vi "Init2DListCtrl.vi"(8 "align":enum16{"Left", "Center", "Right"}(ring), 9 "background color":u32(colorbox)=16777226, 10 "type":enum16{"left frame", "top frame", "content"}(ring), 11 "ArrayRef in":refnum<vi>) -> (3 "ArrayRef out":refnum<vi>)   [LabVIEW 2018, in "Library-Ctrl.lvlib"]
uses:
  Library-Ctrl.lvlib
  <vilib>/Utility/miscctls.llb/LVRowAndColumnTypeDef.ctl
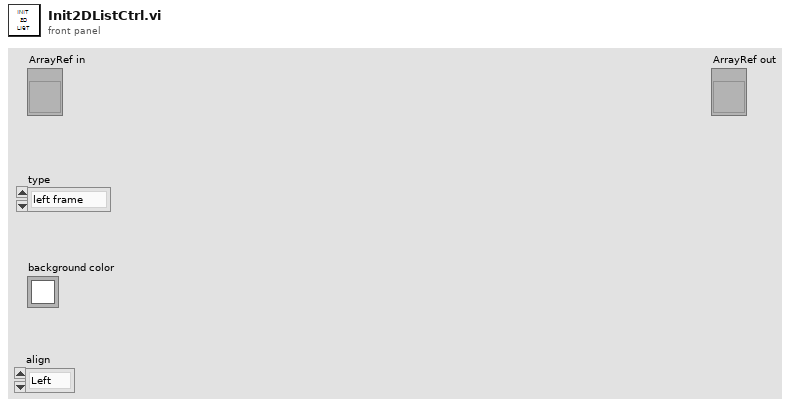
[diagram p1: front panel]
types:
  T1 = typedef "LVRowAndColumnTypeDef.ctl" = cluster{"Row":i32, "Column":i32}
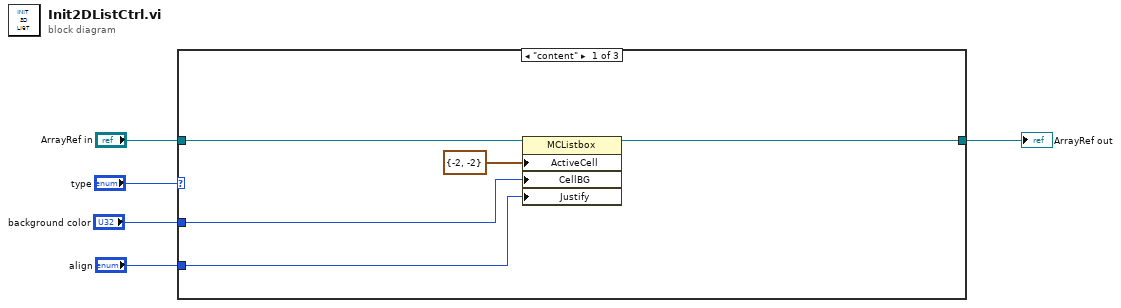
[diagram p0: block diagram]
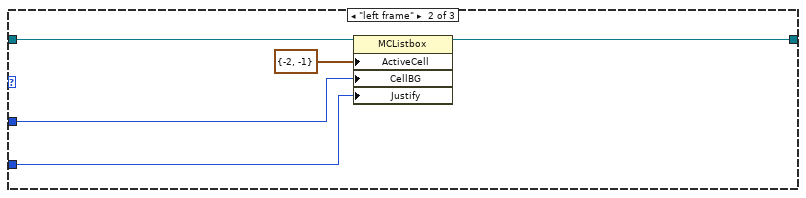
[diagram p2: hidden frame]
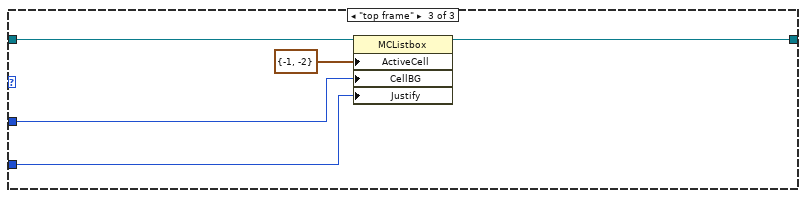
[diagram p3: hidden frame]
diagram:
  n1 = case shown="\"content\"" "type" {
    tunnel: "ArrayRef in" -> [w9 w14 w19]
    tunnel: [w8 w13 w18] -> w4
    tunnel: "background color" -> [w7 w12 w17]
    tunnel: "align" -> [w6 w11 w16]
    frame "content" {
      n2 = property class="MCListbox"(reference=w9, "ActiveCell"=T1 {"Row"=-2, "Column"=-2} ("활성 셀:활성 셀"), "CellBG"=w7, "Justify"=w6) -> (reference out=w8:refnum<vi>)  [unwired: 1 in, 1 out]
    }
    frame "left frame" {
      n3 = property class="MCListbox"(reference=w14, "ActiveCell"=T1 {"Row"=-2, "Column"=-1} ("활성 셀:활성 셀"), "CellBG"=w12, "Justify"=w11) -> (reference out=w13:refnum<vi>)  [unwired: 1 in, 1 out]
    }
    frame "top frame" {
      n4 = property class="MCListbox"(reference=w19, "ActiveCell"=T1 {"Row"=-1, "Column"=-2} ("활성 셀:활성 셀"), "CellBG"=w17, "Justify"=w16) -> (reference out=w18:refnum<vi>)  [unwired: 1 in, 1 out]
    }
  }
  "ArrayRef out" <- w4
